vi "ReadDataFile.vi"(0 "file path (dialog if empty)":path) -> (1 "曲线对应标尺编号":i32[](array[numeric]), 3 "曲线名":string[](array[string]), 4 "通量数据":dbl[][](array[numeric]), 5 "时间间隔":dbl, 6 "P2数据":dbl[][](array[numeric]), 8 "曲线数":i32, 9 "开始时间":timestamp, 10 "反应性数据":dbl[][](array[numeric]), 11 "总时长(s)":dbl, 12 "起止时间":string, 13 "error out":errorcluster, 14 "备注数组":string[](array[string]), 15 "波形簇":cluster{dbl, dbl, dbl[][]})   [LabVIEW 2020]
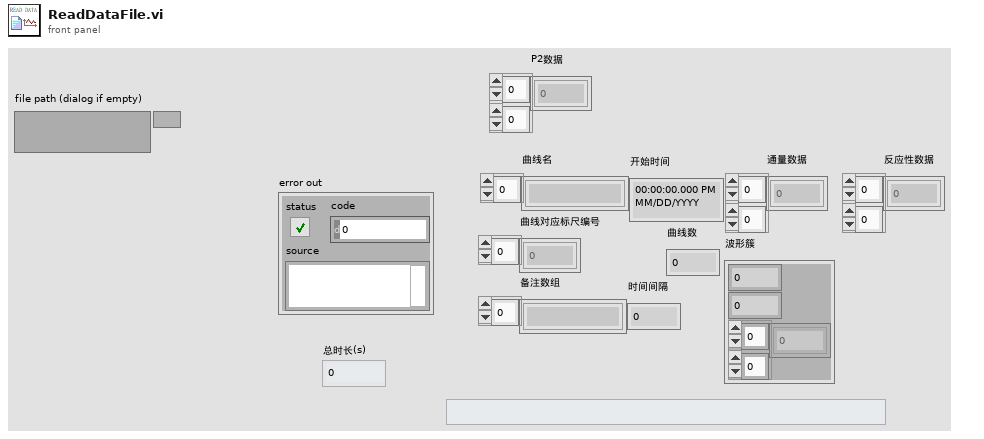
[diagram p1: front panel]
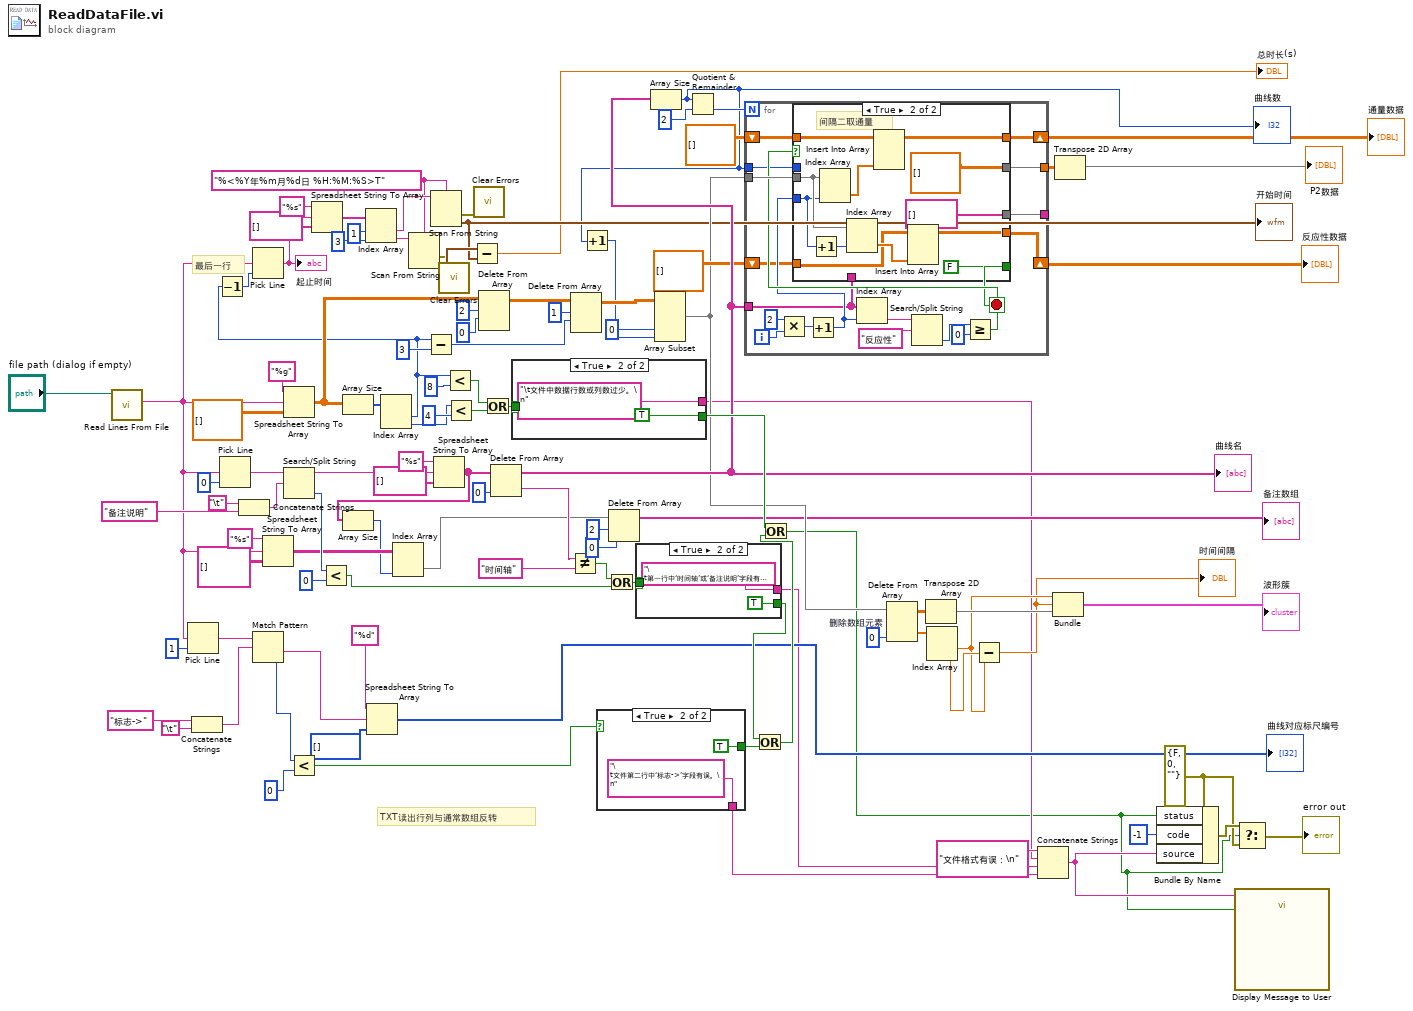
[diagram p0: block diagram]
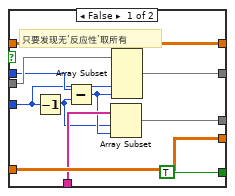
[diagram p2: hidden frame]
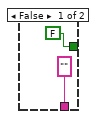
[diagram p3: hidden frame]
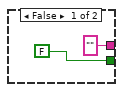
[diagram p4: hidden frame]
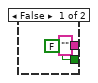
[diagram p5: hidden frame]
diagram:
  w3 = errorcluster {"status"=FALSE, "code"=0, "source"=""} ("error out")
  w26 = "%<%Y年%m月%d日 %H:%M:%S>T" ("格式字符串")
  # "TXT读出行列与通常数组反转"
  # "最后一行"
  n1 = call <vilib>:"Read Lines From File.vi"("file path (dialog if empty)"="file path (dialog if empty)") -> ("line string"=w42:string)  [unwired: 5 in, 3 out]
  n2 = Pick Line(multi-line string=w42, line index=1 ("行索引")) -> (output string=w85:string)  [unwired: 1 in]
  n3 = Concatenate Strings("标志->" ("搜索字符串/字符(-)"), "\t") -> (w82:string)
  n4 = Pick Line(multi-line string=w42, line index=0 ("行索引")) -> (output string=w101:string)  [unwired: 1 in]
  n5 = Concatenate Strings("\t", "备注说明" ("搜索字符串/字符(-)")) -> (w66:string)
  n6 = Match Pattern(string=w85, regular expression=w82) -> (after substring=w79:string, offset past match=w74:i32)  [unwired: 1 in, 2 out]
  n7 = Spreadsheet String To Array ("电子表格字符串至数组转换")(format string="%s" ("format (%.3f)"), spreadsheet string=w42, array type (2D Dbl)=string[][] [] ("添加的数组")) -> (array=w41:string[][])  [unwired: 1 in]
  n8 = Spreadsheet String To Array ("电子表格字符串至数组转换")(format string="%g" ("format (%.3f)"), spreadsheet string=w42, array type (2D Dbl)=dbl[][] [] ("type (empty)")) -> (array=w68:dbl[][])  [unwired: 1 in]
  n9 = Search/Split String(string=w101, search string/char (-)=w66) -> (substring before match=w100:string, offset of match=w99:i32)  [unwired: 1 in, 1 out]
  n10 = Less?(x=w74, y=0) -> (x < y?=w73:bool)
  n11 = Less?(x=w99, y=0) -> (x < y?=w96:bool)
  n12 = Array Size(array=w68) -> (size(s)=w107:i32[])
  n13 = Spreadsheet String To Array ("电子表格字符串至数组转换")(format string="%d" ("format (%.3f)"), spreadsheet string=w79, array type (2D Dbl)=i32[] [] ("添加的数组")) -> (array=→"曲线对应标尺编号":i32[])  [unwired: 1 in]
  n14 = Index Array(array=w107) -> (element #1=w35:i32, element #2=w91:i32)  [unwired: 2 in]
  n15 = Decrement(x=w35) -> (x-1=w36:i32)
  n16 = Pick Line(multi-line string=w42, line index=w36) -> (output string=w34:string)  [unwired: 1 in]
  "起止时间" <- w34
  n17 = Spreadsheet String To Array(format string="%s" ("格式字符串"), spreadsheet string=w34, array type (2D Dbl)=string[] [] ("添加的数组")) -> (array=w31:string[])  [unwired: 1 in]
  n18 = Index Array(array=w31, index #1=1 ("索引"), index #2=3 ("索引")) -> (element #1=w28:string, element #2=w27:string)
  n19 = Scan From String(format string=w26, input string=w27) -> (error out=w21:errorcluster, output 1=w25:timestamp)  [unwired: 3 in, 2 out]
  n20 = Subtract(x=w35, y=3) -> (x-y=w63:i32)
  n21 = Scan From String(format string=w26, input string=w28) -> (error out=w22:errorcluster, output 1=w24:timestamp)  [unwired: 3 in, 2 out]
  "开始时间" <- w24
  n22 = Spreadsheet String To Array ("电子表格字符串至数组转换")(format string="%s" ("format (%.3f)"), spreadsheet string=w100, array type (2D Dbl)=string[] [] ("添加的数组")) -> (array=w40:string[])  [unwired: 1 in]
  n23 = Array Size(array=w40) -> (size(s)=w39:i32)
  n24 = Index Array(array=w41, index (col)=w39) -> (element=w16:string[])  [unwired: 1 in]
  n25 = call <vilib>:"Clear Errors.vi"("error in (no error)"=w21) -> ()  [unwired: 5 in, 2 out]
  n26 = Less?(x=w35, y=8) -> (x < y?=w89:bool)
  n27 = Less?(x=w91, y=4) -> (x < y?=w88:bool)
  n28 = Subtract(x=w25, y=w24) -> (x-y=→"总时长(s)":dbl)
  n29 = call <vilib>:"Clear Errors.vi"("error in (no error)"=w22) -> ()  [unwired: 5 in, 2 out]
  n30 = Delete From Array(array=w68, length=2 ("长度"), index (row)=0 ("索引")) -> (array with subset deleted=w67:dbl[][])  [unwired: 1 in, 1 out]
  n31 = Or(x=w89, y=w88) -> (x .or. y?=w90:bool)
  n32 = Delete From Array(array=w40, index=0 ("索引")) -> (deleted portion=w49:string, array with subset deleted=w57:string[])  [unwired: 1 in]
  "曲线名" <- w57
  n33 = case shown="True" w90 {
    tunnel: w90 -> [_ _]
    tunnel: [FALSE TRUE] -> w87
    tunnel: ["" ("y") "\t文件中数据行数或列数过少。\n" ("y")] -> w8
    frame False {
    }
    frame True {
    }
  }
  n34 = Not Equal?(x=w49, y="时间轴") -> (x != y?=w95:bool)
  n35 = Delete From Array(array=w67, length=1 ("长度"), index (row)=w63) -> (array with subset deleted=w48:dbl[][])  [unwired: 1 in, 1 out]
  n36 = case shown="True" w73 {
    tunnel: [FALSE TRUE] -> w78
    tunnel: ["" ("y") "\t文件第二行中‘标志->’字段有误。\n" ("y")] -> w6
    frame False {
    }
    frame True {
    }
  }
  n37 = Or(x=w95, y=w96) -> (x .or. y?=w94:bool)
  n38 = Delete From Array(array=w16, length=2, index=0) -> (array with subset deleted=→"备注数组":string[])  [unwired: 1 out]
  n39 = case shown="True" w94 {
    tunnel: w94 -> [_ _]
    tunnel: [FALSE TRUE] -> w77
    tunnel: ["" ("y") "\t第一行中‘时间轴’或‘备注说明’字段有误。\n" ("y")] -> w7
    frame False {
    }
    frame True {
    }
  }
  n40 = Array Size(array=w57) -> (size(s)=w20:i32)
  "曲线数" <- w20
  n41 = Increment(x=w20) -> (x+1=w45:i32)
  n42 = Array Subset(array=w48, index (col)=0 ("索引"), length (col)=w45) -> (w47:dbl[][])  [unwired: 2 in]
  n43 = Quotient & Remainder(x=w20, y=2) -> (floor(x/y)=w60:i32)  [unwired: 1 out]
  n44 = for {
    N: w60 -> [_]
    tunnel: w47 -> [w132]
    tunnel: w57 -> [w121]
    shift-right: [w130] -> w58
    shift-left: dbl[][] [] ("type (empty)") -> [w131]
    tunnel: w20 -> [w126]
    tunnel: [w125] -> w59
    shift-right: [w122] -> w52
    shift-left: dbl[][] [] ("type (empty)") -> [w123]
    tunnel: [w120] -> _
    i -> [w138]
    stop <- w127 stop-if-true
    n45 = Multiply(x=2, y=w138) -> (x*y=w124:i32)
    n46 = Increment(x=w124) -> (x+1=w128:i32)
    n47 = Index Array(array=w121, index=w128) -> (element=w136:string)
    n48 = Search/Split String(string=w136, search string/char (-)="反应性" ("搜索字符串/字符(-)")) -> (offset of match=w134:i32)  [unwired: 1 in, 2 out]
    n49 = Greater Or Equal?(x=w134, y=0) -> (x >= y?=w129:bool)
    n50 = case shown="True" w129 {
      tunnel: w132 -> [w147 w156]
      tunnel: w131 -> [w149 w161]
      tunnel: [w149 w159] -> w130
      tunnel: w128 -> [w142 w151]
      tunnel: [TRUE FALSE] -> w127
      tunnel: w126 -> [w146 _]
      tunnel: [w145 dbl[][] [] ("type (empty)")] -> w125
      tunnel: w123 -> [w144 w154]
      tunnel: [w144 w153] -> w122
      tunnel: w121 -> [w143 _]
      tunnel: [w140 string[] []] -> w120
      frame False {
        # "只要发现无‘反应性’取所有"
        n51 = Decrement(x=w142) -> (x-1=w139:i32)
        n52 = Subtract(x=w146, y=w139) -> (x-y=w141:i32)
        n53 = Array Subset(array=w143, index=w139, length=w141) -> (w140:string[])
        n54 = Array Subset(array=w147, index (col)=w142, length (col)=w141) -> (w145:dbl[][])  [unwired: 2 in]
      }
      frame True {
        # "间隔二取通量"
        n55 = Increment(x=w151) -> (x+1=w152:i32)
        n56 = Index Array(array=w156, index (col)=w151) -> (element=w160:dbl[])  [unwired: 1 in]
        n57 = Index Array(array=w156, index (col)=w152) -> (element=w155:dbl[])  [unwired: 1 in]
        n58 = Insert Into Array(array=w161, new element=w160) -> (w159:dbl[][])  [unwired: 2 in]
        n59 = Insert Into Array(array=w154, new element=w155) -> (w153:dbl[][])  [unwired: 2 in]
      }
    }
  }
  "通量数据" <- w58
  "反应性数据" <- w52
  n60 = Or(x=w77, y=w78) -> (x .or. y?=w76:bool)
  n61 = Or(x=w87, y=w76) -> (x .or. y?=w1:bool)
  n62 = Delete From Array "删除数组元素"(array=w47, index (col)=0 ("禁用的索引 (列)")) -> (deleted portion=w51:dbl[], array with subset deleted=w55:dbl[][])  [unwired: 2 in]
  n63 = Transpose 2D Array(2D array=w55) -> (transposed array=w19:dbl[][])
  n64 = Index Array(array=w51) -> (element #1=w17:dbl, element #2=w50:dbl)  [unwired: 2 in]
  n65 = Subtract(x=w50, y=w17) -> (x-y=w11:dbl)
  "时间间隔" <- w11
  n66 = Concatenate Strings("文件格式有误：\n" ("string"), w8, w7, w6) -> (w2:string)
  n67 = Bundle(w17, w11, w19) -> (→"波形簇":cluster{dbl, dbl, dbl[][]})  [unwired: 1 in]
  n68 = Transpose 2D Array(2D array=w59) -> (transposed array=→"P2数据":dbl[][])
  n69 = Bundle By Name(cluster=w3, "status"=w1, "code"=-1, "source"=w2) -> (w4:errorcluster)
  n70 = call "Display Message to User"("Enable"=w1, "Message"=w2) -> ()  [unwired: 8 in, 2 out]
  n71 = Select(t=w4, s=w1, f=w3) -> (s? t:f=→"error out":errorcluster)
